vi "Setup VI for Screen With custom size.vi"(7 "Position":enum16{"Top Left", "Centre"}(ring), 8 "Error In":errorcluster, 9 "Width":i16, 10 "Height":i16, 11 "This VI":refnum<vi>) -> (0 "Error Out":errorcluster, 3 "VI Ref Out":refnum<vi>)   [LabVIEW 2014]
uses:
  <vilib>/Utility/miscctls.llb/LVPointTypeDef.ctl
  <vilib>/Utility/miscctls.llb/LVRectTypeDef.ctl
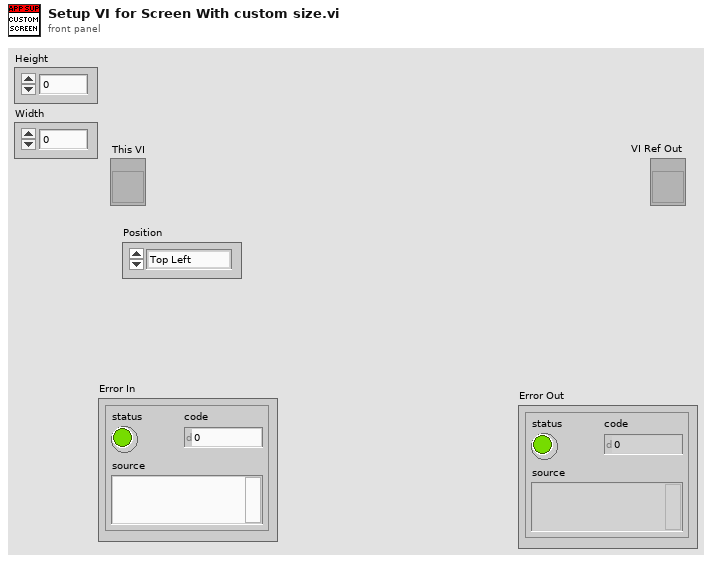
[diagram p1: front panel]
types:
  T1 = typedef "LVRectTypeDef.ctl" = cluster{"Left":i16, "Top":i16, "Right":i16, "Bottom":i16}
  T2 = typedef "LVPointTypeDef.ctl" = cluster{"Horizontal":i16, "Vertical":i16}
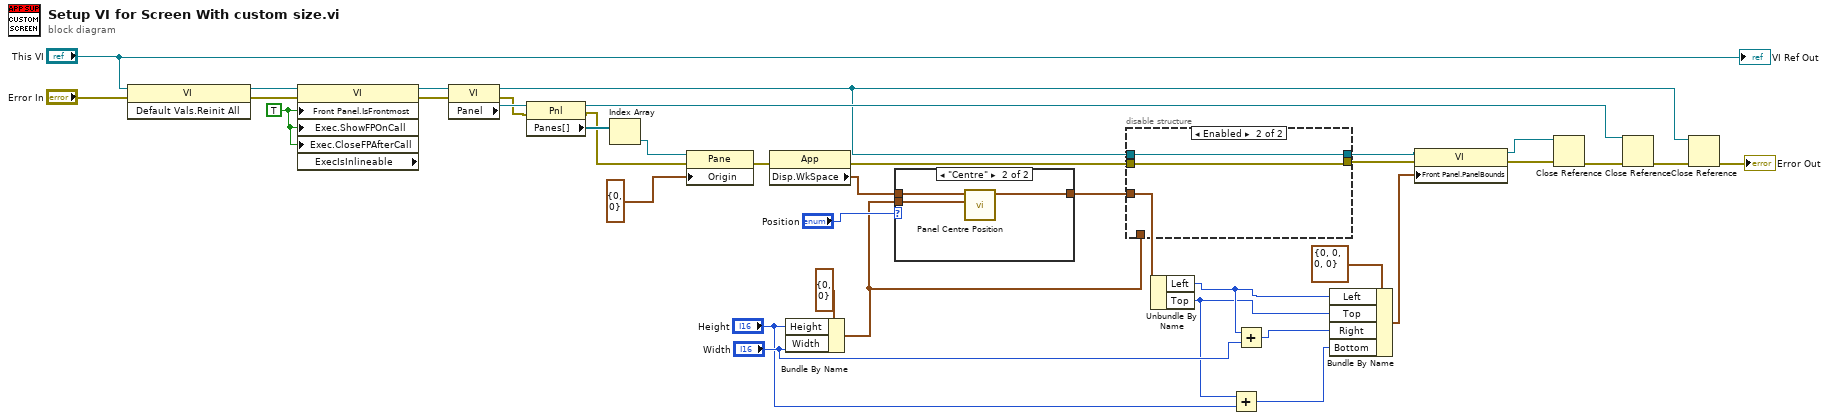
[diagram p0: block diagram]
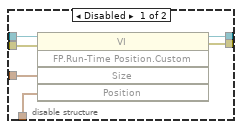
[diagram p2: hidden frame]
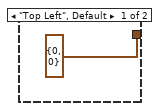
[diagram p3: hidden frame]
diagram:
  w20 = TRUE ("Front Panel Window:Is Frontmost")
  n1 = invoke class="VI" method="Default Vals.Reinit All"(reference="This VI", error in="Error In") -> (reference out=w24:refnum<vi>, error out=w21:errorcluster)  [unwired: 1 in, 1 out]
  n2 = property on="Property Node" class="VI" props=["Front Panel.IsFrontmost", "Exec.ShowFPOnCall", "Exec.CloseFPAfterCall", "ExecIsInlineable"](reference=w24, error in=w21, "Front Panel.IsFrontmost"=w20, "Exec.ShowFPOnCall"=w20, "Exec.CloseFPAfterCall"=w20) -> (reference out=w23:refnum<vi>, error out=w22:errorcluster)  [unwired: 1 out]
  n3 = property on="Property Node" class="VI"(reference=w23, error in=w22) -> (reference out=w25:refnum<vi>, error out=w31:errorcluster, "Panel"=w35:refnum<vi>)
  n4 = property on="Property Node" class="Pnl"(reference=w35, error in=w31) -> (reference out=w28:refnum<vi>, error out=w30:errorcluster, "Panes[]"=w34:refnum<vi>[])
  n5 = Index Array(array=w34) -> (element=w33:refnum<vi>)  [unwired: 1 in]
  n6 = property on="Property Node" class="Pane"(reference=w33, error in=w30, "Origin"=T2 {"Horizontal"=0, "Vertical"=0}) -> (error out=w19:errorcluster)  [unwired: 1 out]
  n7 = property class="App"(error in=w19) -> (error out=w18:errorcluster, "Disp.WkSpace"=w17:T1)  [unwired: 1 in, 1 out]
  n8 = Bundle By Name(cluster=cluster{"Height":i16, "Width":i16} {"Height"=0, "Width"=0} ("Panel size"), "Height"="Height", "Width"="Width") -> (w14:cluster{"Height":i16, "Width":i16})
  n9 = case shown="\"Centre\"" "Position" {
    tunnel: w17 -> [_ w41]
    tunnel: w14 -> [_ w40]
    tunnel: [cluster{"Top":i16, "Left":i16} {"Top"=0, "Left"=0} ("Position") w39] -> w7
    frame "Top Left", Default {
    }
    frame "Centre" {
      n10 = call "Panel Centre Position.vi"("Panel size"=w40, "Monitor Bounds"=w41) -> ("Position"=w39:cluster{"Top":i16, "Left":i16})  [unwired: 9 in]
    }
  }
  n11 = disable-structure shown="Enabled" {
    disable-tunnel: w25 -> [w47 w48]
    disable-tunnel: w18 -> [w46 w49]
    disable-tunnel: w14 -> [w45 _]
    disable-tunnel: [w44 w48] -> w11
    disable-tunnel: [w43 w49] -> w10
    disable-tunnel: w7 -> [w42 _]
    frame Disabled {
      n12 = invoke class="VI" method="FP.Run-Time Position.Custom"(reference=w47, error in=w46, "Size"=w42, "Position"=w45) -> (reference out=w44:refnum<vi>, error out=w43:errorcluster)  [unwired: 1 in, 3 out]
    }
    frame Enabled {
    }
  }
  n13 = Unbundle By Name(w7) -> ("Left"=w6:i16, "Top"=w3:i16)
  n14 = Add(x=w3, y="Height") -> (x+y=w1:i16)
  n15 = Add(x=w6, y="Width") -> (x+y=w4:i16)
  n16 = Bundle By Name(cluster=T1 {"Left"=0, "Top"=0, "Right"=0, "Bottom"=0} ("Front Panel Window:Panel Bounds"), "Left"=w6, "Top"=w3, "Right"=w4, "Bottom"=w1) -> (w8:T1)
  n17 = property class="VI"(reference=w11, error in=w10, "Front Panel.PanelBounds"=w8) -> (reference out=w12:refnum<vi>, error out=w13:errorcluster)
  n18 = Close Reference(reference=w12, error in (no error)=w13) -> (error out=w29:errorcluster)
  n19 = Close Reference(reference=w28, error in (no error)=w29) -> (error out=w27:errorcluster)
  n20 = Close Reference(reference=w25, error in (no error)=w27) -> (error out=→"Error Out":errorcluster)
  "VI Ref Out" <- "This VI"
